vi "Read Results from processing.vi"(8 "error in":errorcluster, 11 "My Awesome Control Modules runtime in":refnum<class "My Awesome Control Modules runtime.lvclass">) -> (0 "error out":errorcluster, 2 "Results from processing":T1, 3 "My Awesome Control Modules runtime out":refnum<class "My Awesome Control Modules runtime.lvclass">)   [LabVIEW 2013, in "My Awesome Control Modules runtime.lvclass"]
uses:
  My Awesome Control Modules runtime.lvclass
  configuration/result data indices.ctl
  configuration/My Awesome Control Modules configuration.lvclass
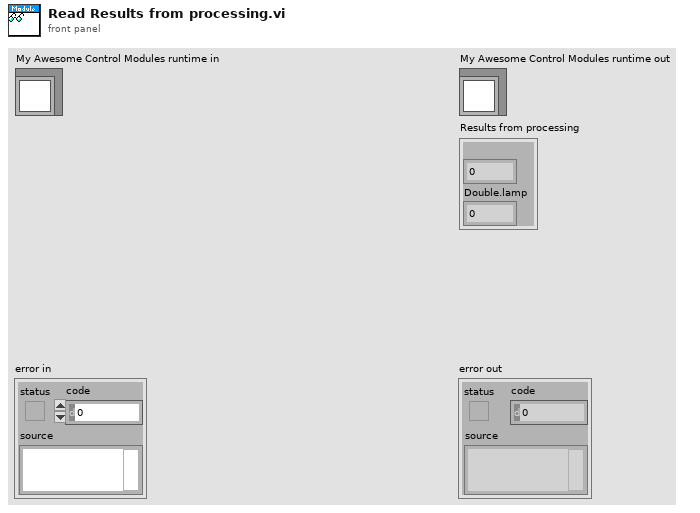
[diagram p1: front panel]
types:
  T1 = typedef "My Awesome Control Modules configuration.lvclass/result data indices.ctl" = cluster{"Double.fan":i32, "Double.lamp":i32}
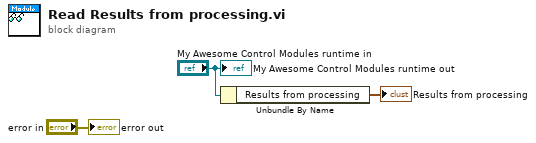
[diagram p0: block diagram]
diagram:
  n1 = Unbundle By Name("My Awesome Control Modules runtime in") -> ("Results from processing"=→"Results from processing":T1)
  "error out" <- "error in"
  "My Awesome Control Modules runtime out" <- "My Awesome Control Modules runtime in"
